vi "AB_RW_Project_Source_ExportedVI.vi"(7 "action":T4, 8 "error in (no error)":errorcluster, 9 "index in":i32, 10 "dataSource in":T1, 11 "buildObject":T3) -> (0 "error out":errorcluster, 1 "index out":i32, 2 "dataSource out":T1, 3 "buildObject out":T3)   [LabVIEW 2020]
doc: "Reads and writes the data to the object property bag."
uses:
  <resource>/Framework/Providers/API/ItemRef.ctl
  <vilib>/AppBuilder/RW_Project/AB_RW_Project_PropBag_Action.ctl
  <vilib>/AppBuilder/RW_Project/AB_RW_Project_Source_ExportedVI_Data_New.ctl
  <vilib>/AppBuilder/ABAPI Dist VI Proto Info New.ctl
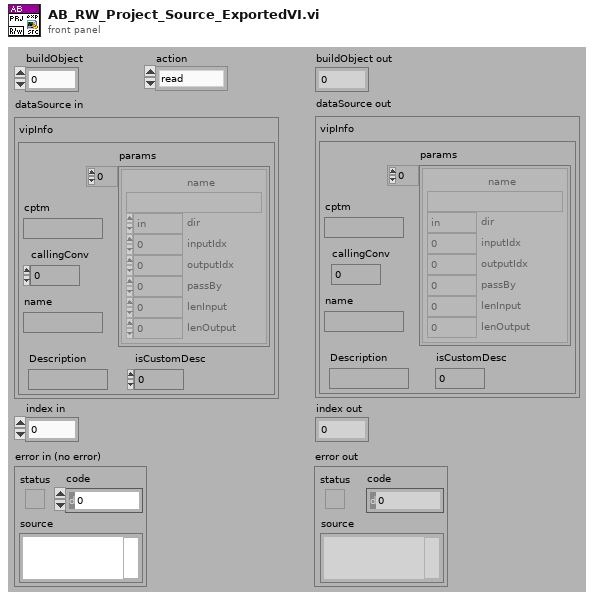
[diagram p1: front panel]
types:
  T1 = typedef "AB_RW_Project_Source_ExportedVI_Data_New.ctl" = cluster{"vipInfo":T2}
  T2 = typedef "ABAPI Dist VI Proto Info New.ctl" = cluster{"cptm":string, "params":cluster{"name":string, "dir":enum32{"in", "out", "in/out", "length", "error-out"}, "inputIdx":i32, "outputIdx":i32, "passBy":i32, "lenInput":i32, "lenOutput":i32}[], "callingConv":i32, "name":string, "Description":string, "isCustomDesc":i32}
  T3 = typedef "ItemRef.ctl" = u64
  T4 = typedef "AB_RW_Project_PropBag_Action.ctl" = enum16{"read", "write", "clear", "readPrevious", "writePrevious", "clearPrevious"}
  T5 = cluster{"name":string, "dir":enum32{"in", "out", "in/out", "length", "error-out"}, "inputIdx":i32, "outputIdx":i32, "passBy":i32, "lenInput":i32, "lenOutput":i32}
  T6 = cluster{"name":string, "dir":enum32{"in", "out", "in/out", "length", "error-out"}, "inputIdx":i32, "outputIdx":i32, "passBy":i32, "lenInput":i32, "lenOutput":i32}[]
  T7 = enum32{"in", "out", "in/out", "length", "error-out"}
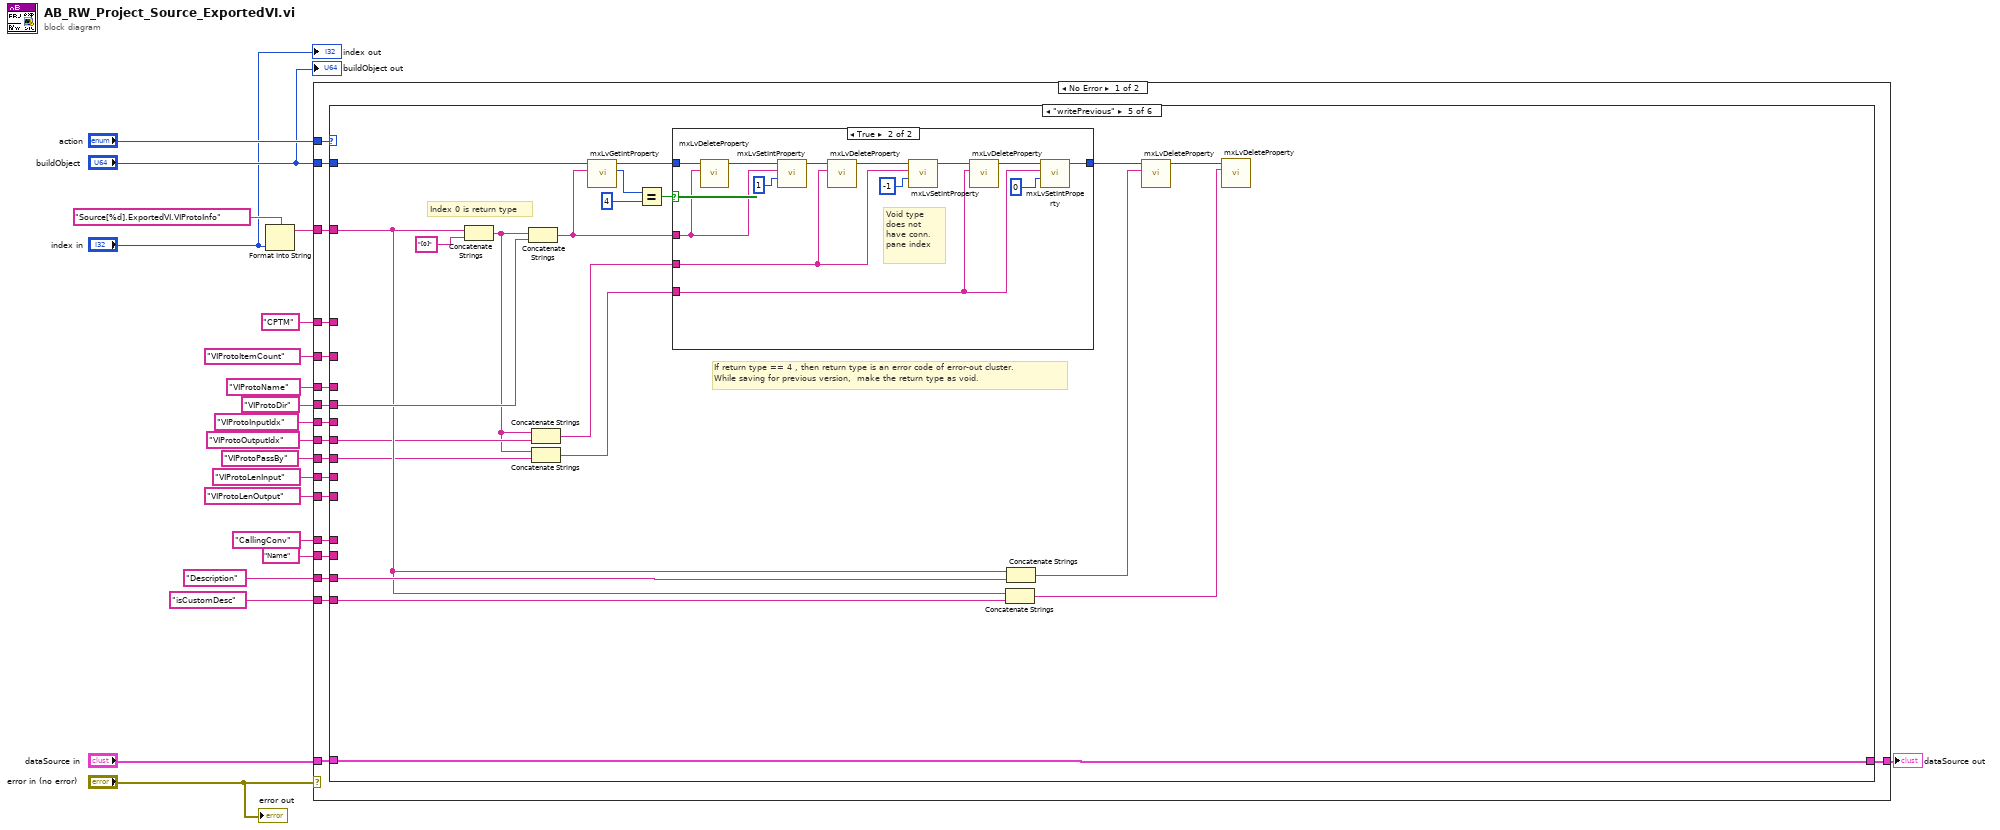
[diagram p0: block diagram]
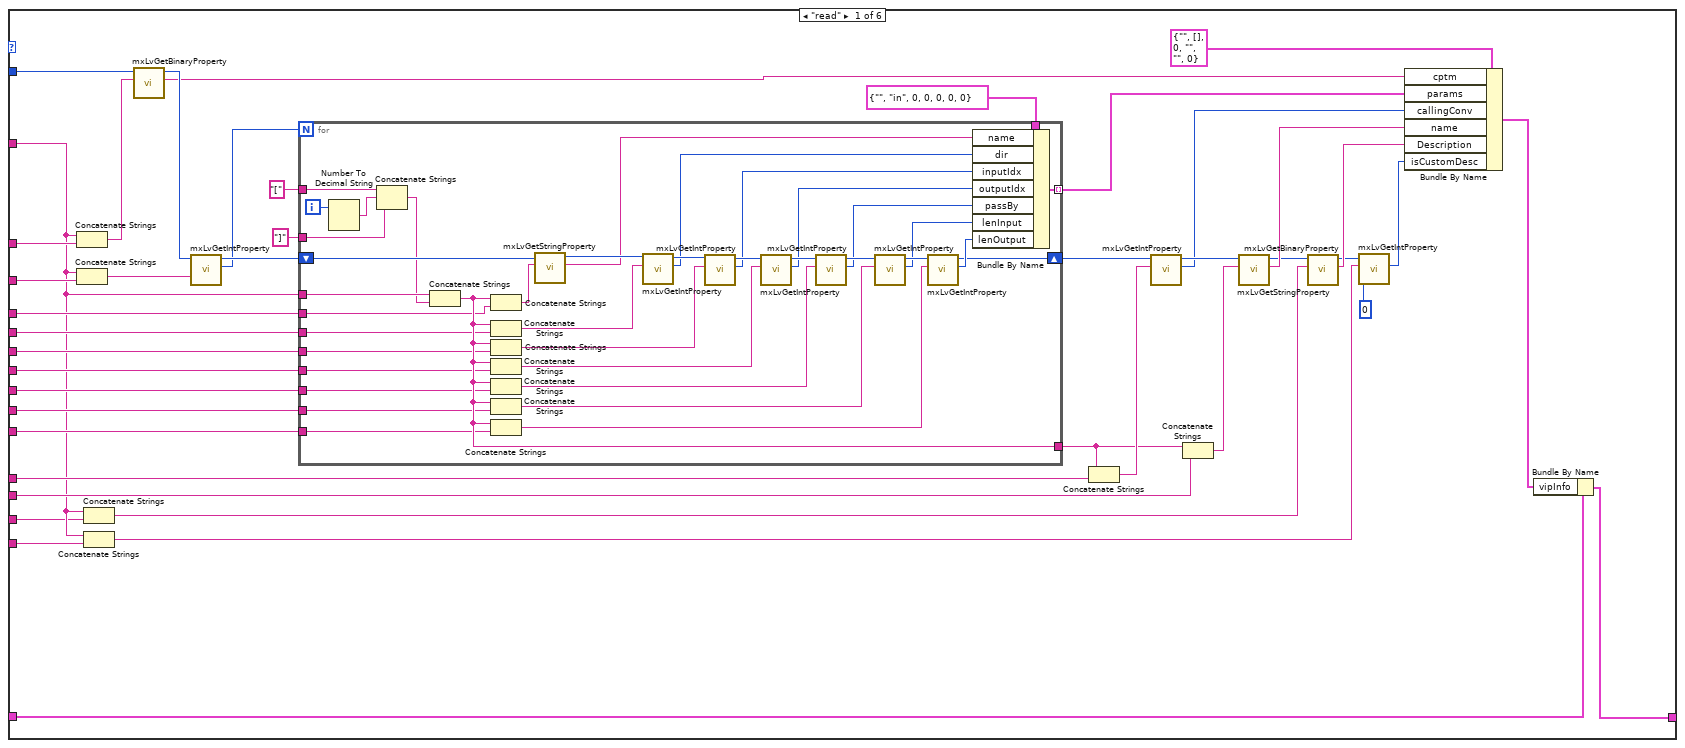
[diagram p2: hidden frame]
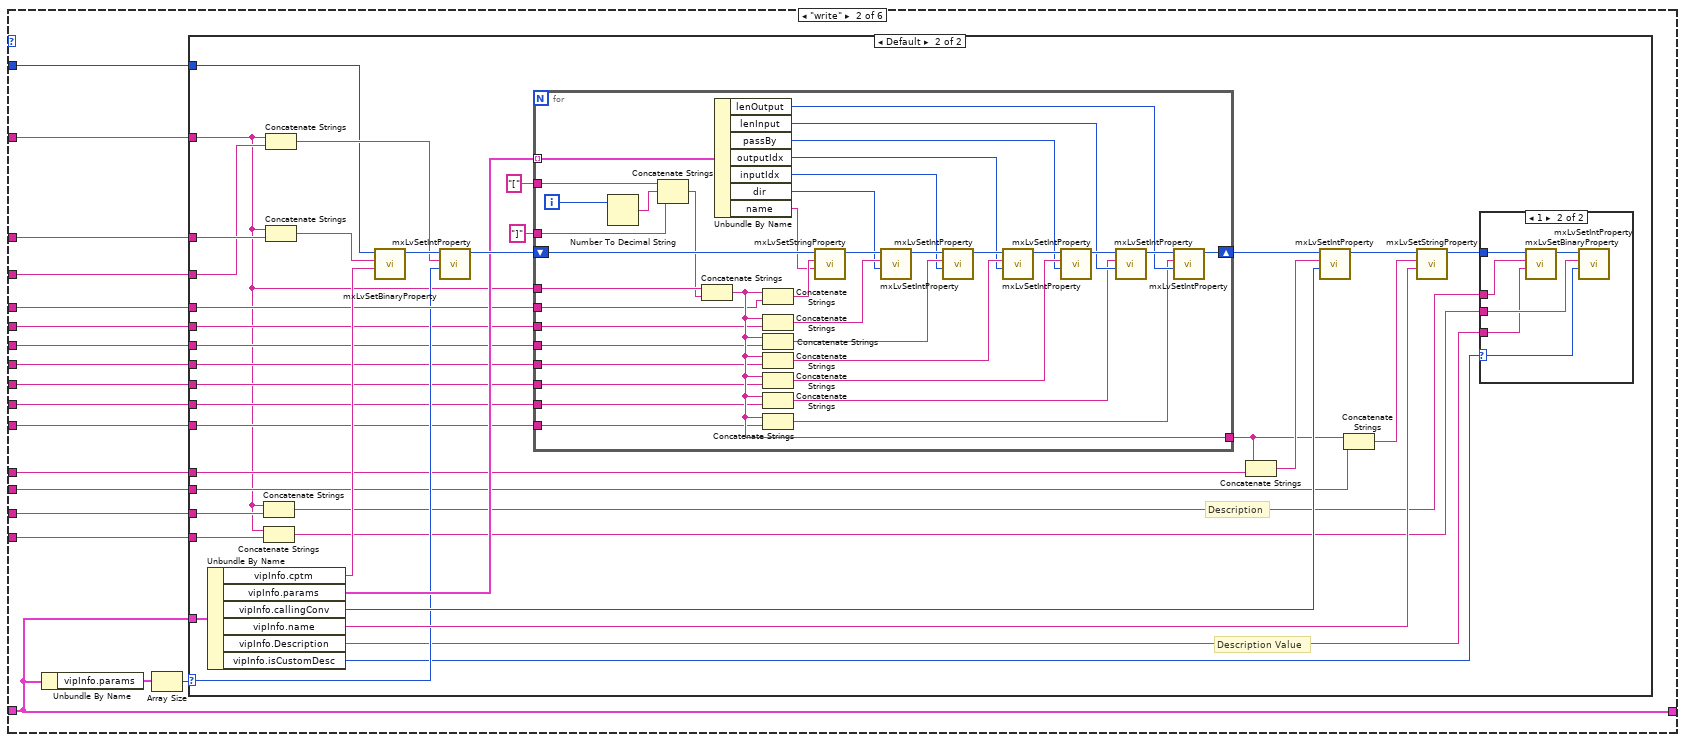
[diagram p3: hidden frame]
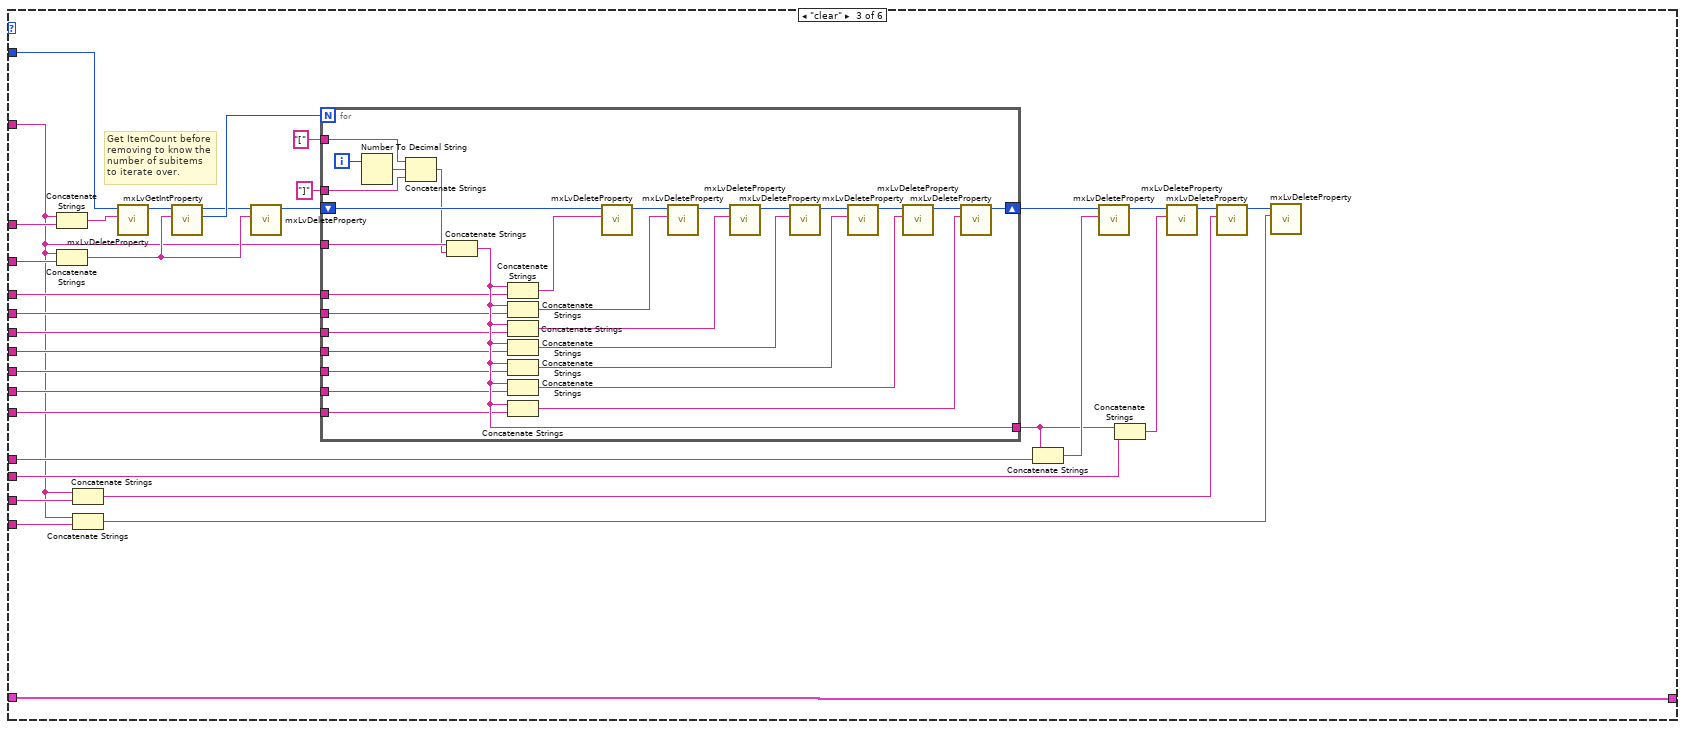
[diagram p6: hidden frame]
diagram:
  n1 = Format Into String(format string="Source[%d].ExportedVI.VIProtoInfo", "index in") -> (resulting string=w19:string)  [unwired: 2 in, 1 out]
  n2 = case shown="No Error" "error in (no error)" {
    tunnel: "action" -> [w39 _]
    tunnel: "dataSource in" -> [w38 w318]
    tunnel: w19 -> [w37 _]
    tunnel: "buildObject" -> [w36 _]
    tunnel: [w35 w318] -> w14
    tunnel: "CPTM" -> [w34 _]
    tunnel: "VIProtoItemCount" -> [w33 _]
    tunnel: "VIProtoName" ("string") -> [w32 _]
    tunnel: "VIProtoDir" ("string") -> [w31 _]
    tunnel: "VIProtoInputIdx" ("string") -> [w30 _]
    tunnel: "VIProtoOutputIdx" ("string") -> [w29 _]
    tunnel: "VIProtoPassBy" ("string") -> [w28 _]
    tunnel: "VIProtoLenInput" ("string") -> [w27 _]
    tunnel: "VIProtoLenOutput" ("string") -> [w26 _]
    tunnel: "CallingConv" -> [w25 _]
    tunnel: "Name" -> [w24 _]
    tunnel: "Description" -> [w23 _]
    tunnel: "isCustomDesc" -> [w22 _]
    frame No Error {
      n3 = case shown="\"writePrevious\"" w39 {
        tunnel: w36 -> [w80 w136 w249 _ w293 _]
        tunnel: w38 -> [w82 w131 w251 w281 w302 w317]
        tunnel: w37 -> [w51 w137 w223 _ w294 _]
        tunnel: [w81 w131 w251 w281 w302 w317] -> w35
        tunnel: w34 -> [w62 w134 w250 _ _ _]
        tunnel: w33 -> [w61 w133 w248 _ _ _]
        tunnel: w32 -> [w60 w135 w234 _ _ _]
        tunnel: w31 -> [w59 w130 w233 _ w296 _]
        tunnel: w30 -> [w58 w129 w232 _ _ _]
        tunnel: w29 -> [w57 w128 w231 _ w285 _]
        tunnel: w28 -> [w56 w127 w230 _ w286 _]
        tunnel: w27 -> [w55 w126 w229 _ _ _]
        tunnel: w26 -> [w54 w125 w228 _ _ _]
        tunnel: w25 -> [w53 w124 w226 _ _ _]
        tunnel: w24 -> [w52 w123 w227 _ _ _]
        tunnel: w23 -> [w50 w121 w224 _ w301 _]
        tunnel: w22 -> [w49 w122 w225 _ w300 _]
        frame "read" {
          n4 = Concatenate Strings(w51, w62) -> (w78:string)
          n5 = Concatenate Strings(w51, w61) -> (w74:string)
          n6 = Concatenate Strings(w51, w50) -> (w44:string)
          n7 = Concatenate Strings(w51, w49) -> (w48:string)
          n8 = call <resource>:"mxLvGetBinaryProperty.vi"("Tag"=w78, "Item"=w80) -> ("Value"=w63:string, "Item"=w75:T3)  [unwired: 7 in, 1 out]
          n9 = call <resource>:"mxLvGetIntProperty.vi"("Tag"=w74, "Item"=w75) -> ("Value"=w68:i32, "Item"=w73:T3)  [unwired: 7 in, 1 out]
          n10 = for {
            N: w68 -> [_]
            tunnel: "[" -> [w119]
            tunnel: "]" -> [w118]
            tunnel: w51 -> [w113]
            tunnel: [w100] -> w69
            tunnel: T5 {"name"="", "dir"=enum."in", "inputIdx"=0, "outputIdx"=0, "passBy"=0, "lenInput"=0, "lenOutput"=0} -> [w99]
            tunnel: [w91] -> w41 mode=indexing
            shift-right: [w90] -> w64
            shift-left: w73 -> [w116]
            tunnel: w60 -> [w89]
            tunnel: w59 -> [w88]
            tunnel: w58 -> [w87]
            tunnel: w57 -> [w86]
            tunnel: w56 -> [w85]
            tunnel: w55 -> [w84]
            tunnel: w54 -> [w83]
            i -> [w117]
            n11 = Number To Decimal String(number=w117) -> (decimal integer string=w120:string)  [unwired: 1 in]
            n12 = Concatenate Strings(w119, w120, w118) -> (w112:string)
            n13 = Concatenate Strings(w113, w112) -> (w100:string)
            n14 = Concatenate Strings(w100, w89) -> (w115:string)
            n15 = Concatenate Strings(w100, w88) -> (w111:string)
            n16 = Concatenate Strings(w100, w87) -> (w110:string)
            n17 = Concatenate Strings(w100, w86) -> (w104:string)
            n18 = Concatenate Strings(w100, w85) -> (w103:string)
            n19 = Concatenate Strings(w100, w84) -> (w102:string)
            n20 = Concatenate Strings(w100, w83) -> (w101:string)
            n21 = call <resource>:"mxLvGetStringProperty.vi"("Tag"=w115, "Item"=w116) -> ("Value"=w98:string, "Item"=w114:T3)  [unwired: 7 in, 1 out]
            n22 = call <resource>:"mxLvGetIntProperty.vi"("Tag"=w111, "Item"=w114) -> ("Value"=w97:i32, "Item"=w109:T3)  [unwired: 7 in, 1 out]
            n23 = call <resource>:"mxLvGetIntProperty.vi"("Tag"=w110, "Item"=w109) -> ("Value"=w96:i32, "Item"=w108:T3)  [unwired: 7 in, 1 out]
            n24 = call <resource>:"mxLvGetIntProperty.vi"("Tag"=w104, "Item"=w108) -> ("Value"=w95:i32, "Item"=w107:T3)  [unwired: 7 in, 1 out]
            n25 = call <resource>:"mxLvGetIntProperty.vi"("Tag"=w103, "Item"=w107) -> ("Value"=w94:i32, "Item"=w106:T3)  [unwired: 7 in, 1 out]
            n26 = call <resource>:"mxLvGetIntProperty.vi"("Tag"=w102, "Item"=w106) -> ("Value"=w93:i32, "Item"=w105:T3)  [unwired: 7 in, 1 out]
            n27 = call <resource>:"mxLvGetIntProperty.vi"("Tag"=w101, "Item"=w105) -> ("Value"=w92:i32, "Item"=w90:T3)  [unwired: 7 in, 1 out]
            n28 = Bundle By Name(cluster=w99, "name"=w98, "dir"=w97, "inputIdx"=w96, "outputIdx"=w95, "passBy"=w94, "lenInput"=w93, "lenOutput"=w92) -> (w91:T5)
          }
          n29 = Concatenate Strings(w69, w53) -> (w76:string)
          n30 = call <resource>:"mxLvGetIntProperty.vi"("Tag"=w76, "Item"=w64) -> ("Value"=w66:i32, "Item"=w70:T3)  [unwired: 7 in, 1 out]
          n31 = Concatenate Strings(w69, w52) -> (w77:string)
          n32 = call <resource>:"mxLvGetStringProperty.vi"("Tag"=w77, "Item"=w70) -> ("Value"=w65:string, "Item"=w45:T3)  [unwired: 7 in, 1 out]
          n33 = call <resource>:"mxLvGetBinaryProperty.vi"("Tag"=w44, "Item"=w45) -> ("Value"=w43:string, "Item"=w42:T3)  [unwired: 7 in, 1 out]
          n34 = call <resource>:"mxLvGetIntProperty.vi"("Default Value (0)"=0, "Tag"=w48, "Item"=w42) -> ("Value"=w47:i32)  [unwired: 6 in, 2 out]
          n35 = Bundle By Name(cluster=T2 {"cptm"="", "params"=[], "callingConv"=0, "name"="", "Description"="", "isCustomDesc"=0} ("vipInfo in"), "cptm"=w63, "params"=w41, "callingConv"=w66, "name"=w65, "Description"=w43, "isCustomDesc"=w47) -> (w79:T2)
          n36 = Bundle By Name(cluster=w82, "vipInfo"=w79) -> (w81:T1)
        }
        frame "write" {
          n37 = Unbundle By Name(w131) -> ("vipInfo.params"=w138:T6)
          n38 = Array Size(array=w138) -> (size(s)=w132:i32)
          n39 = case shown="Default" w132 {
            selector: w132 -> [_ w155]
            tunnel: w136 -> [_ w160]
            tunnel: w131 -> [_ w159]
            tunnel: w137 -> [_ w144]
            tunnel: w135 -> [_ w158]
            tunnel: w134 -> [_ w157]
            tunnel: w133 -> [_ w156]
            tunnel: w130 -> [_ w154]
            tunnel: w129 -> [_ w153]
            tunnel: w128 -> [_ w152]
            tunnel: w127 -> [_ w151]
            tunnel: w126 -> [_ w150]
            tunnel: w125 -> [_ w149]
            tunnel: w124 -> [_ w148]
            tunnel: w123 -> [_ w147]
            tunnel: w122 -> [_ w146]
            tunnel: w121 -> [_ w145]
            frame 0 {
              # "If default, then don't write anything out."
            }
            frame Default {
              # "Description Value"
              # "Description"
              n40 = Unbundle By Name(w159) -> ("vipInfo.cptm"=w174:string, "vipInfo.params"=w166:T6, "vipInfo.callingConv"=w170:i32, "vipInfo.name"=w171:string, "vipInfo.Description"=w140:string, "vipInfo.isCustomDesc"=w141:i32)
              n41 = Concatenate Strings(w144, w145) -> (w143:string)
              n42 = Concatenate Strings(w144, w146) -> (w142:string)
              n43 = Concatenate Strings(w144, w156) -> (w168:string)
              n44 = Concatenate Strings(w144, w157) -> (w175:string)
              n45 = call <resource>:"mxLvSetBinaryProperty.vi"("Value"=w174, "Tag"=w175, "Item"=w160) -> ("Item"=w169:T3)  [unwired: 7 in, 1 out]
              n46 = call <resource>:"mxLvSetIntProperty.vi"("Value (0)"=w155, "Tag"=w168, "Item"=w169) -> ("Item"=w167:T3)  [unwired: 7 in, 1 out]
              n47 = for {
                tunnel: w166 -> [w218] mode=indexing
                tunnel: "[" -> [w216]
                tunnel: "]" -> [w215]
                tunnel: w144 -> [w209]
                tunnel: [w190] -> w161
                shift-right: [w189] -> w163
                shift-left: w167 -> [w213]
                tunnel: w158 -> [w188]
                tunnel: w154 -> [w187]
                tunnel: w153 -> [w186]
                tunnel: w152 -> [w185]
                tunnel: w151 -> [w184]
                tunnel: w150 -> [w183]
                tunnel: w149 -> [w182]
                i -> [w214]
                n48 = Number To Decimal String(number=w214) -> (decimal integer string=w217:string)  [unwired: 1 in]
                n49 = Concatenate Strings(w216, w217, w215) -> (w208:string)
                n50 = Concatenate Strings(w209, w208) -> (w190:string)
                n51 = Unbundle By Name(w218) -> ("lenOutput"=w192:i32, "lenInput"=w194:i32, "passBy"=w195:i32, "outputIdx"=w196:i32, "inputIdx"=w203:i32, "dir"=w206:T7, "name"=w211:string)
                n52 = Concatenate Strings(w190, w188) -> (w212:string)
                n53 = Concatenate Strings(w190, w187) -> (w207:string)
                n54 = Concatenate Strings(w190, w186) -> (w205:string)
                n55 = Concatenate Strings(w190, w185) -> (w198:string)
                n56 = Concatenate Strings(w190, w184) -> (w197:string)
                n57 = Concatenate Strings(w190, w183) -> (w193:string)
                n58 = Concatenate Strings(w190, w182) -> (w191:string)
                n59 = call <resource>:"mxLvSetStringProperty.vi"("Value (\"\")"=w211, "Tag"=w212, "Item"=w213) -> ("Item"=w210:T3)  [unwired: 7 in, 1 out]
                n60 = call <resource>:"mxLvSetIntProperty.vi"("Value (0)"=w206, "Tag"=w207, "Item"=w210) -> ("Item"=w204:T3)  [unwired: 7 in, 1 out]
                n61 = call <resource>:"mxLvSetIntProperty.vi"("Value (0)"=w203, "Tag"=w205, "Item"=w204) -> ("Item"=w202:T3)  [unwired: 7 in, 1 out]
                n62 = call <resource>:"mxLvSetIntProperty.vi"("Value (0)"=w196, "Tag"=w198, "Item"=w202) -> ("Item"=w201:T3)  [unwired: 7 in, 1 out]
                n63 = call <resource>:"mxLvSetIntProperty.vi"("Value (0)"=w195, "Tag"=w197, "Item"=w201) -> ("Item"=w200:T3)  [unwired: 7 in, 1 out]
                n64 = call <resource>:"mxLvSetIntProperty.vi"("Value (0)"=w194, "Tag"=w193, "Item"=w200) -> ("Item"=w199:T3)  [unwired: 7 in, 1 out]
                n65 = call <resource>:"mxLvSetIntProperty.vi"("Value (0)"=w192, "Tag"=w191, "Item"=w199) -> ("Item"=w189:T3)  [unwired: 7 in, 1 out]
              }
              n66 = Concatenate Strings(w161, w148) -> (w172:string)
              n67 = call <resource>:"mxLvSetIntProperty.vi"("Value (0)"=w170, "Tag"=w172, "Item"=w163) -> ("Item"=w162:T3)  [unwired: 7 in, 1 out]
              n68 = Concatenate Strings(w161, w147) -> (w173:string)
              n69 = call <resource>:"mxLvSetStringProperty.vi"("Value (\"\")"=w171, "Tag"=w173, "Item"=w162) -> ("Item"=w139:T3)  [unwired: 7 in, 1 out]
              n70 = case shown="1" w141 {
                selector: w141 -> [_ w180]
                tunnel: w142 -> [_ w181]
                tunnel: w143 -> [_ w178]
                tunnel: w140 -> [_ w177]
                tunnel: w139 -> [_ w179]
                frame 0, Default {
                }
                frame 1 {
                  n71 = call <resource>:"mxLvSetBinaryProperty.vi"("Value"=w177, "Tag"=w178, "Item"=w179) -> ("Item"=w176:T3)  [unwired: 7 in, 1 out]
                  n72 = call <resource>:"mxLvSetIntProperty.vi"("Value (0)"=w180, "Tag"=w181, "Item"=w176) -> ()  [unwired: 7 in, 2 out]
                }
              }
            }
          }
        }
        frame "clear" {
          # "Get ItemCount before removing to know the number of subitems to iterate over."
          n73 = Concatenate Strings(w223, w250) -> (w247:string)
          n74 = Concatenate Strings(w223, w248) -> (w235:string)
          n75 = Concatenate Strings(w223, w224) -> (w221:string)
          n76 = Concatenate Strings(w223, w225) -> (w222:string)
          n77 = call <resource>:"mxLvDeleteProperty.vi"("Tag"=w247, "Item"=w249) -> ("Item"=w237:T3)  [unwired: 8 in, 1 out]
          n78 = call <resource>:"mxLvGetIntProperty.vi"("Tag"=w235, "Item"=w237) -> ("Value"=w238:i32, "Item"=w236:T3)  [unwired: 7 in, 1 out]
          n79 = call <resource>:"mxLvDeleteProperty.vi"("Tag"=w235, "Item"=w236) -> ("Item"=w244:T3)  [unwired: 8 in, 1 out]
          n80 = for {
            N: w238 -> [_]
            tunnel: "[" -> [w279]
            tunnel: "]" -> [w278]
            tunnel: w223 -> [w273]
            tunnel: [w260] -> w239
            shift-right: [w259] -> w241
            shift-left: w244 -> [w276]
            tunnel: w234 -> [w258]
            tunnel: w233 -> [w257]
            tunnel: w232 -> [w256]
            tunnel: w231 -> [w255]
            tunnel: w230 -> [w254]
            tunnel: w229 -> [w253]
            tunnel: w228 -> [w252]
            i -> [w277]
            n81 = Number To Decimal String(number=w277) -> (decimal integer string=w280:string)  [unwired: 1 in]
            n82 = Concatenate Strings(w279, w280, w278) -> (w272:string)
            n83 = Concatenate Strings(w273, w272) -> (w260:string)
            n84 = Concatenate Strings(w260, w258) -> (w275:string)
            n85 = Concatenate Strings(w260, w257) -> (w271:string)
            n86 = Concatenate Strings(w260, w256) -> (w270:string)
            n87 = Concatenate Strings(w260, w255) -> (w264:string)
            n88 = Concatenate Strings(w260, w254) -> (w263:string)
            n89 = Concatenate Strings(w260, w253) -> (w262:string)
            n90 = Concatenate Strings(w260, w252) -> (w261:string)
            n91 = call <resource>:"mxLvDeleteProperty.vi"("Tag"=w275, "Item"=w276) -> ("Item"=w274:T3)  [unwired: 8 in, 1 out]
            n92 = call <resource>:"mxLvDeleteProperty.vi"("Tag"=w271, "Item"=w274) -> ("Item"=w269:T3)  [unwired: 8 in, 1 out]
            n93 = call <resource>:"mxLvDeleteProperty.vi"("Tag"=w270, "Item"=w269) -> ("Item"=w268:T3)  [unwired: 8 in, 1 out]
            n94 = call <resource>:"mxLvDeleteProperty.vi"("Tag"=w264, "Item"=w268) -> ("Item"=w267:T3)  [unwired: 8 in, 1 out]
            n95 = call <resource>:"mxLvDeleteProperty.vi"("Tag"=w263, "Item"=w267) -> ("Item"=w266:T3)  [unwired: 8 in, 1 out]
            n96 = call <resource>:"mxLvDeleteProperty.vi"("Tag"=w262, "Item"=w266) -> ("Item"=w265:T3)  [unwired: 8 in, 1 out]
            n97 = call <resource>:"mxLvDeleteProperty.vi"("Tag"=w261, "Item"=w265) -> ("Item"=w259:T3)  [unwired: 8 in, 1 out]
          }
          n98 = Concatenate Strings(w239, w226) -> (w245:string)
          n99 = call <resource>:"mxLvDeleteProperty.vi"("Tag"=w245, "Item"=w241) -> ("Item"=w240:T3)  [unwired: 8 in, 1 out]
          n100 = Concatenate Strings(w239, w227) -> (w246:string)
          n101 = call <resource>:"mxLvDeleteProperty.vi"("Tag"=w246, "Item"=w240) -> ("Item"=w220:T3)  [unwired: 8 in, 1 out]
          n102 = call <resource>:"mxLvDeleteProperty.vi"("Tag"=w221, "Item"=w220) -> ("Item"=w219:T3)  [unwired: 8 in, 1 out]
          n103 = call <resource>:"mxLvDeleteProperty.vi"("Tag"=w222, "Item"=w219) -> ()  [unwired: 8 in, 2 out]
        }
        frame "readPrevious" {
        }
        frame "writePrevious" {
          # "Index 0 is return type"
          # "If return type == 4 , then return type is an error code of error-out cluster.\nWhile saving for previous version,  make the return type as void."
          n104 = Concatenate Strings(w294, "[0]" ("string")) -> (w284:string)
          n105 = Concatenate Strings(w284, w296) -> (w287:string)
          n106 = Concatenate Strings(w284, w285) -> (w283:string)
          n107 = Concatenate Strings(w284, w286) -> (w282:string)
          n108 = call <resource>:"mxLvGetIntProperty.vi"("Tag"=w287, "Item"=w293) -> ("Value"=w292:i32, "Item"=w289:T3)  [unwired: 7 in, 1 out]
          n109 = Equal?(x=w292, y=4) -> (x = y?=w290:bool)
          n110 = case shown="True" w290 {
            tunnel: [w303 w306] -> w288
            tunnel: w289 -> [w303 w316]
            tunnel: w287 -> [_ w314]
            tunnel: w283 -> [_ w309]
            tunnel: w282 -> [_ w305]
            frame False {
            }
            frame True {
              # "Void type\ndoes not  \nhave conn.\npane index"
              n111 = call <resource>:"mxLvDeleteProperty.vi"("Tag"=w314, "Item"=w316) -> ("Item"=w315:T3)  [unwired: 8 in, 1 out]
              n112 = call <resource>:"mxLvSetIntProperty.vi"("Value (0)"=1, "Tag"=w314, "Item"=w315) -> ("Item"=w311:T3)  [unwired: 7 in, 1 out]
              n113 = call <resource>:"mxLvDeleteProperty.vi"("Tag"=w309, "Item"=w311) -> ("Item"=w310:T3)  [unwired: 8 in, 1 out]
              n114 = call <resource>:"mxLvSetIntProperty.vi"("Value (0)"=-1, "Tag"=w309, "Item"=w310) -> ("Item"=w307:T3)  [unwired: 7 in, 1 out]
              n115 = call <resource>:"mxLvDeleteProperty.vi"("Tag"=w305, "Item"=w307) -> ("Item"=w308:T3)  [unwired: 8 in, 1 out]
              n116 = call <resource>:"mxLvSetIntProperty.vi"("Value (0)"=0, "Tag"=w305, "Item"=w308) -> ("Item"=w306:T3)  [unwired: 7 in, 1 out]
            }
          }
          n117 = Concatenate Strings(w294, w300) -> (w297:string)
          n118 = Concatenate Strings(w294, w301) -> (w299:string)
          n119 = call <resource>:"mxLvDeleteProperty.vi"("Tag"=w299, "Item"=w288) -> ("Item"=w298:T3)  [unwired: 8 in, 1 out]
          n120 = call <resource>:"mxLvDeleteProperty.vi"("Tag"=w297, "Item"=w298) -> ()  [unwired: 8 in, 2 out]
        }
        frame "clearPrevious" {
        }
      }
    }
    frame Error {
    }
  }
  "dataSource out" <- w14
  "error out" <- "error in (no error)"
  "buildObject out" <- "buildObject"
  "index out" <- "index in"
